vi "Phone-check-login.vi"(4 "Boolean":bool, 6 "MAIL:":string, 7 "NAME:":string, 9 "MOBILE:":string, 10 "LAST NAME:":string, 11 "Boolean in":refnum<vi>) -> (1 "number":dbl[](array[numeric]), 2 "Boolean 2":bool, 3 "WARNING":bool, 5 "Array":string[](array[string]))   [LabVIEW 2016]
panel:
  out "sts":bool
  out "Info_data":string
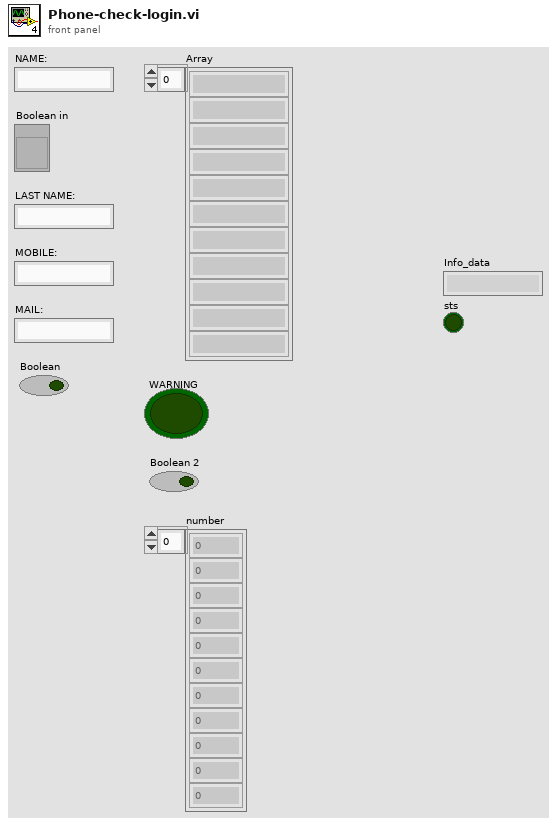
[diagram p1: front panel]
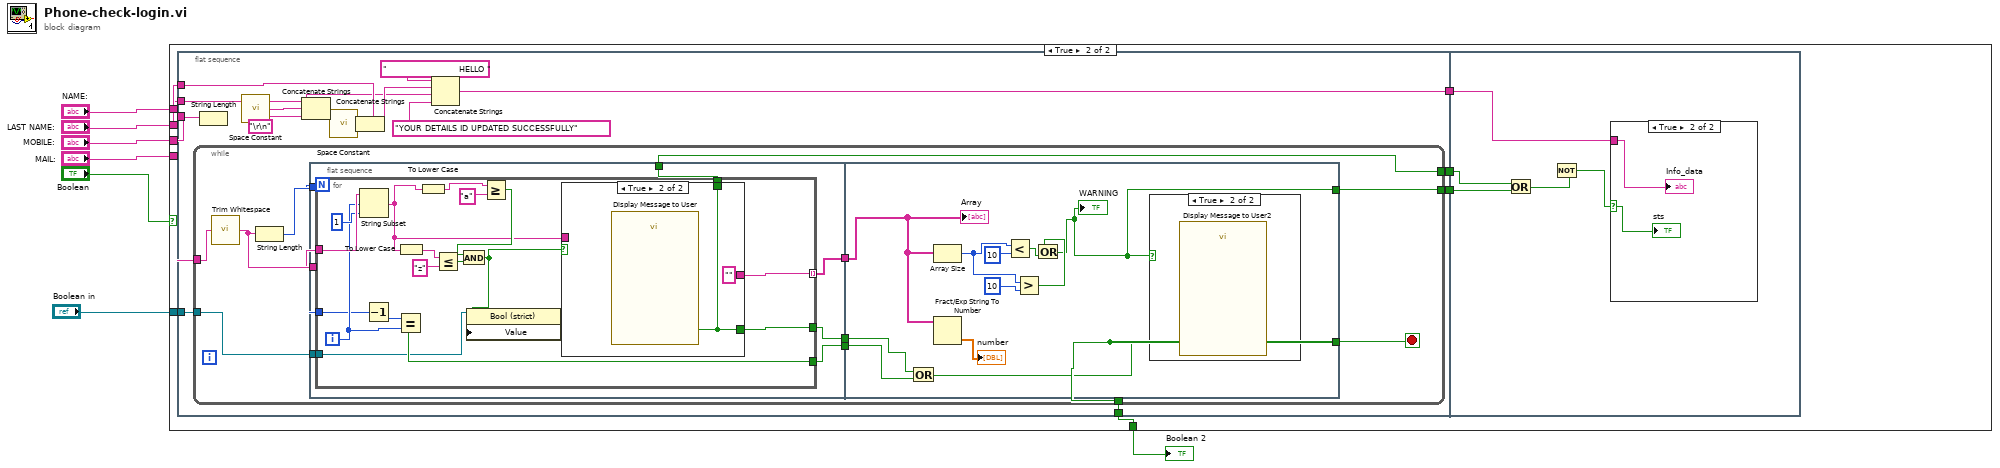
[diagram p0: block diagram]
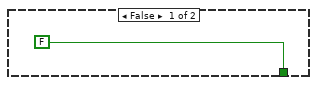
[diagram p2: hidden frame]
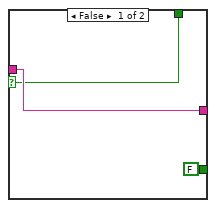
[diagram p3: hidden frame]
diagram:
  n1 = case shown="True" "Boolean" {
    tunnel: "NAME:" -> [_ w16]
    tunnel: "LAST NAME:" -> [_ w15]
    tunnel: "MOBILE:" -> [_ w14]
    tunnel: "MAIL:" -> [_ _]
    tunnel: [FALSE w13] -> w6
    tunnel: "Boolean in" -> [_ w9]
    frame False {
    }
    frame True {
      n2 = flat-sequence {
        tunnel: w16 -> [w29]
        tunnel: w15 -> [w25]
        tunnel: w14 -> [w22]
        tunnel: [w20] -> w13
        tunnel: [w21] -> w12
        tunnel: [w19] -> w11
        tunnel: [w18] -> w10
        tunnel: w9 -> [w17]
        tunnel: w12 -> [w83]
        tunnel: w11 -> [w86]
        tunnel: w10 -> [w87]
        frame #0 {
          n3 = while {
            tunnel: w22 -> [w41]
            tunnel: [w35] -> w20
            tunnel: [w34] -> w19
            tunnel: [w33] -> w18
            tunnel: w17 -> [w32]
            stop <- w35 stop-if-true
            n4 = call <vilib>:"Trim Whitespace.vi"("string"=w41) -> ("trimmed string"=w40:string)  [unwired: 1 in]
            n5 = String Length(string=w40) -> (length=w39:i32)
            n6 = flat-sequence {
              tunnel: w40 -> [w48]
              tunnel: w39 -> [w46]
              tunnel: [w47] -> w38
              tunnel: [w45] -> w37
              tunnel: [w44] -> w36
              tunnel: [w43] -> w33
              tunnel: w32 -> [w42]
              tunnel: w38 -> [w79]
              tunnel: w37 -> [w82]
              tunnel: w36 -> [w81]
              tunnel: [w80] -> w35
              tunnel: [w72] -> w34
              frame #0 {
                n7 = for {
                  N: w46 -> [_]
                  tunnel: w48 -> [w66]
                  tunnel: [w60] -> w47 mode=indexing
                  tunnel: [w59] -> w45
                  tunnel: w46 -> [w56]
                  tunnel: [w55] -> w44
                  tunnel: [w50] -> w43
                  tunnel: w42 -> [w49]
                  i -> [w58]
                  n8 = String Subset(string=w66, offset (0)=w58, length (rest)=1 ("length (rest)")) -> (substring=w53:string)
                  n9 = Decrement(x=w56) -> (x-1=w57:i32)
                  n10 = Equal?(x=w57, y=w58) -> (x = y?=w55:bool)
                  n11 = To Lower Case(string=w53) -> (all lower case string=w52:string)
                  n12 = To Lower Case(string=w53) -> (all lower case string=w54:string)
                  n13 = Less Or Equal?(x=w52, y="z") -> (x <= y?=w61:bool)
                  n14 = Greater Or Equal?(x=w54, y="a") -> (x >= y?=w62:bool)
                  n15 = And(x=w62, y=w61) -> (x .and. y?=w51:bool)
                  n16 = property class="Bool (strict)"(reference=w49, "Value"=w51) -> ()  [unwired: 1 in, 2 out]
                  n17 = case shown="True" w51 {
                    selector: w51 -> [w67 _]
                    tunnel: w53 -> [w69 _]
                    tunnel: [w69 "" ("trimmed string")] -> w60
                    tunnel: [FALSE ("OK") w70] -> w59
                    tunnel: [w67 w70] -> w50
                    frame False {
                    }
                    frame True {
                      n18 = call "Display Message to User"() -> ("OK"=w70:bool)  [unwired: 10 in, 1 out]
                    }
                  }
                }
              }
              frame #1 {
                n19 = Or(x=w82, y=w81) -> (x .or. y?=w80:bool)
                n20 = Array Size(array=w79) -> (size(s)=w74:i32)
                n21 = Fract/Exp String To Number(string=w79) -> (number=→"number":dbl[])  [unwired: 3 in, 1 out]
                n22 = Less?(x=w74, y=10) -> (x < y?=w77:bool)
                n23 = Greater?(x=w74, y=10) -> (0:w76:bool)
                n24 = Or(x=w76, y=w77) -> (x .or. y?=w72:bool)
                "WARNING" <- w72
                n25 = case shown="True" w72 {
                  frame False {
                  }
                  frame True {
                    n26 = call "Display Message to User2"() -> ()  [unwired: 10 in, 2 out]
                  }
                }
                "Array" <- w79
              }
            }
          }
          n27 = String Length(string=w22) -> ()  [unwired: 1 out]
          n28 = call <vilib>:"Space Constant.vi"() -> ("String"=w26:string)
          n29 = Concatenate Strings(w25, w26, "\r\n") -> (w24:string)
          n30 = call <vilib>:"Space Constant.vi"() -> ("String"=w28:string)
          n31 = Concatenate Strings(w29, w28) -> (w27:string)
          n32 = Concatenate Strings("                        HELLO " ("string"), w27, w24, "YOUR DETAILS ID UPDATED SUCCESSFULLY" ("string")) -> (w21:string)
        }
        frame #1 {
          n33 = Or(x=w87, y=w86) -> (x .or. y?=w85:bool)
          n34 = Not(x=w85) -> (.not. x?=w84:bool)
          n35 = case shown="True" w84 {
            selector: w84 -> [_ w88]
            tunnel: w83 -> [_ w89]
            frame False {
            }
            frame True {
              "Info_data" <- w89
              "sts" <- w88
            }
          }
        }
      }
    }
  }
  "Boolean 2" <- w6
